vi "CheckCRC.vi"(8 "CRC Increment":u32=256, 9 "Special Value":u32=3328, 10 "AND Value":u32=65280, 11 "CRC In":u32) -> (3 "CRC Out":u32)   [LabVIEW 2012, in "Sierra-M100.lvlib"]
doc: "This VI checks to make sure the CRC is correct before sending it to the mass flow controller. There are reserved bytes that the CRC cannot contain."
uses:
  Sierra-M100.lvlib
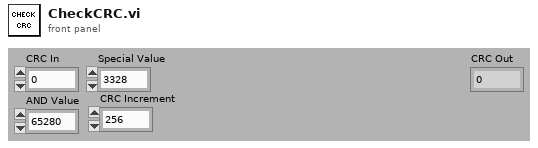
[diagram p1: front panel]
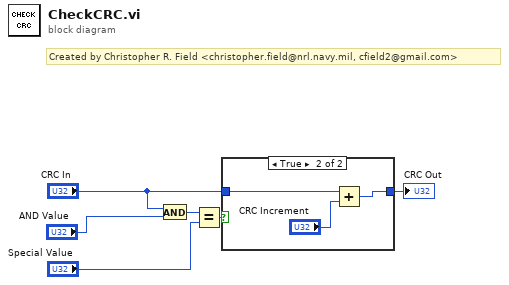
[diagram p0: block diagram]
diagram:
  # "Created by Christopher R. Field <christopher.field@nrl.navy.mil, cfield2@gmail.com>"
  n1 = And(x="CRC In", y="AND Value") -> (x .and. y?=w4:u32)
  n2 = Equal?(x=w4, y="Special Value") -> (x = y?=w6:bool)
  n3 = case shown="True" w6 {
    tunnel: "CRC In" -> [w7 w10]
    tunnel: [w7 w8] -> w1
    frame False {
    }
    frame True {
      n4 = Add(x=w10, y="CRC Increment") -> (x+y=w8:u32)
    }
  }
  "CRC Out" <- w1
